vi "PH_gentec_M-Link.range 2 string.vi"(1 "Range":T1 items=["1f", "3f", "10f", "30f", "100f", "300f", "1p", "3p", "10p", "30p", "100p", "300p", "1n", "3n", "10n", "30n", "100n", "300n", "1u", "3u", "10u", "30u", "100u", "300u", "1m", "3m", "10m", "30m", "100m", "300m", "1", "3", "10", "30", "100", "300", "1K", "3K", "10K", "30K", "100K", "300K", "1M", "3M", "10M", "30M", "100M", "300M"]) -> (0 "Range as string":string)   [LabVIEW 2014, in "PH_gentec_M-Link.lvlib"]
doc: "This VI gives the range out as string."
uses:
  PH_gentec_M-Link.lvlib
  instr.lib/Gentec-M-Link/Driver/Type Defs/gentec-M-Link.Range.ctl
  instr.lib/Gentec-M-Link/gentec-M-Link - Driver.lvlib
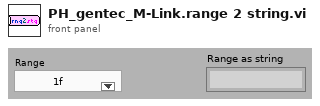
[diagram p1: front panel]
types:
  T1 = typedef "gentec-M-Link - Driver.lvlib/gentec-M-Link.Range.ctl" = u16
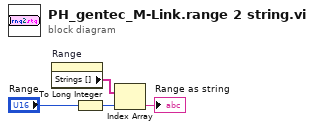
[diagram p0: block diagram]
diagram:
  n1 = property on="Range" class="Ring (strict)"() -> ("Strings []"=w4:string[])  [unwired: 2 in, 2 out]
  n2 = To Long Integer(number="Range") -> (32bit integer=w2:i32)
  n3 = Index Array(array=w4, index=w2) -> (element=→"Range as string":string)
